vi "正弦波转换为方波.vi"() -> ()   [LabVIEW 2012]
uses:
  <vilib>/Analysis/NI_AALBase.lvlib
panel:
  out "正弦波转换为方波":dbl[][](graph)
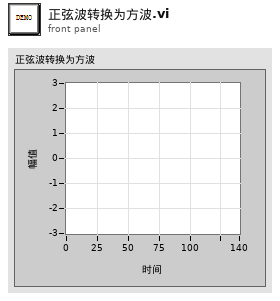
[diagram p1: front panel]
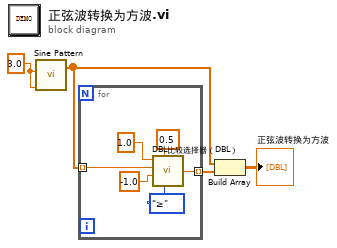
[diagram p0: block diagram]
diagram:
  w1 = 3.0 ("cycles")
  n1 = call <vilib>:"Sine Pattern.vi"("cycles"=w1, "amplitude"=w1) -> ("Sinusoidal Pattern"=w4:dbl[])  [unwired: 2 in, 1 out]
  n2 = for {
    tunnel: w4 -> [w10] mode=indexing
    tunnel: [w5] -> w3 mode=indexing
    n3 = call "DBL比较选择器（DBL）.vi"("A"=1.0, "阙值"=0.5, "信号"=w10, "B"=-1.0, "模式"=enum16{"≠", "＝", "＞", "≥", "＜", "≤"}."≥") -> ("输出"=w5:dbl)  [unwired: 3 in]
  }
  n4 = Build Array(w4, w3) -> (→"正弦波转换为方波":dbl[][])
